vi "Quit LabVIEW if Executable.vi"   [LabVIEW 2010]
doc: "Checks the current path to this VI to see if it is called as part of an executable. If so, the \"Quit LabVIEW\" VI is called.\n\nsupport@labjack.com\nwww.labjack.com\n6/17/2001"
panel:
  # "Checks the current path to this VI to see if it\nis called as part of an executable.  If so, the\n\"Quit LabVIEW\" VI is called.\n\nsupport@labjack.com\nwww.labjack.com\n6/17/2001"
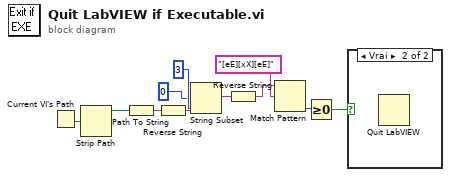
[diagram p0: block diagram]
diagram:
  n1 = Current VI's Path() -> (path=w11:path)
  n2 = Strip Path(path=w11) -> (stripped path=w2:path)  [unwired: 1 out]
  n3 = Path To String(path=w2) -> (string=w10:string)
  n4 = Reverse String(1:w10) -> (0:w9:string)
  n5 = String Subset(string=w9, offset (0)=0, length (rest)=3 ("length")) -> (substring=w6:string)
  n6 = Reverse String(1:w6) -> (0:w5:string)
  n7 = Match Pattern(string=w5, regular expression="[eE][xX][eE]") -> (offset past match=w3:i32)  [unwired: 1 in, 3 out]
  n8 = Greater Or Equal To 0?(x=w3) -> (x >= 0?=w1:bool)
  n9 = case shown="Vrai" w1 {
    frame False {
    }
    frame True {
      n10 = Quit LabVIEW() -> ()  [unwired: 1 in]
    }
  }
